vi "dht11.vi"() -> ()   [LabVIEW 2021]
panel:
  in  "Reset":bool
  out "HUMIDITY":dbl(knob) scale=0.0..100.0
  out "Thermometer":dbl(slide) scale=0.0..100.0
  in  "FAN":bool
  in  "PUMP":bool
  in  "VISA resource name":refnum<visa-resource-name>
  in  "stop":bool
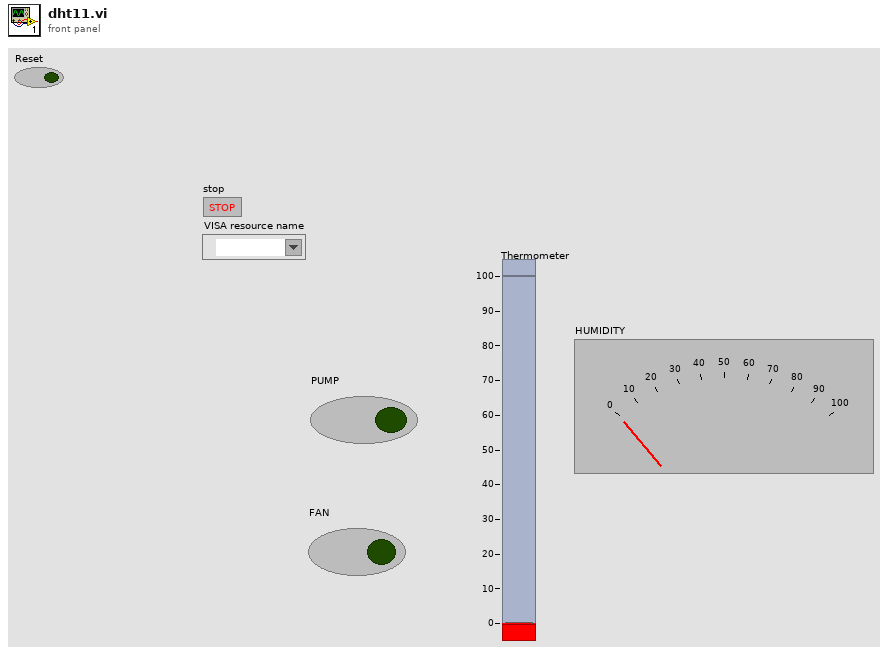
[diagram p1: front panel]
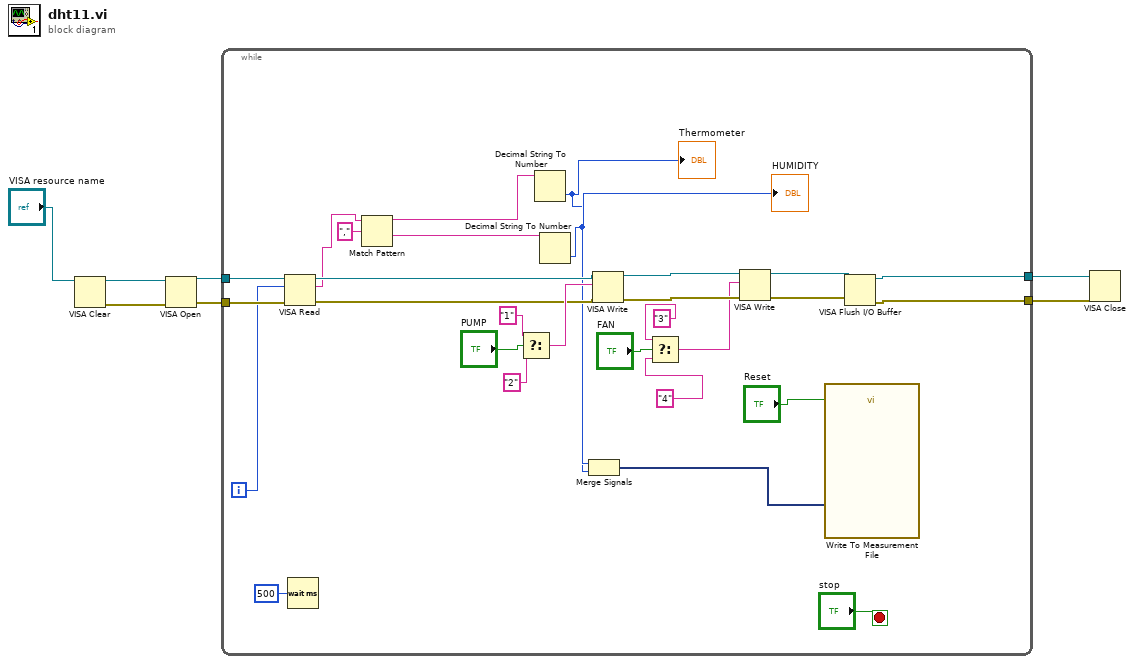
[diagram p0: block diagram]
diagram:
  n1 = VISA Clear(VISA resource name="VISA resource name") -> (VISA resource name out=w7:refnum<visa-resource-name>, error out=w6:errorcluster)  [unwired: 1 in]
  n2 = VISA Open(error in (no error)=w6, VISA resource name=w7) -> (VISA resource name=w5:refnum<visa-resource-name>, error out=w4:errorcluster)  [unwired: 3 in]
  n3 = while {
    tunnel: w5 -> [w36]
    tunnel: w4 -> [w35]
    tunnel: [w34] -> w3
    tunnel: [w33] -> w2
    i -> [w32]
    stop <- "stop" stop-if-true
    n4 = VISA Read(VISA resource name=w36, byte count=w32, error in (no error)=w35) -> (VISA resource name out=w17:refnum<visa-resource-name>, read buffer=w15:string, error out=w16:errorcluster)  [unwired: 1 out]
    n5 = Wait (ms)(milliseconds to wait=u32 500) -> ()  [unwired: 1 out]
    n6 = Match Pattern(string=w15, regular expression=",") -> (before substring=w13:string, after substring=w12:string)  [unwired: 1 in, 2 out]
    n7 = Select(t="1", s="PUMP", f="2") -> (s? t:f=w27:string)
    n8 = Decimal String To Number(string=w13) -> (number=w10:i32)  [unwired: 2 in, 1 out]
    "Thermometer" <- w10
    n9 = Decimal String To Number(string=w12) -> (number=w11:i32)  [unwired: 2 in, 1 out]
    "HUMIDITY" <- w11
    n10 = Merge Signals(w11, w10) -> (w9:dynamicdata)
    n11 = VISA Write(VISA resource name=w17, write buffer=w27, error in (no error)=w16) -> (VISA resource name out=w26:refnum<visa-resource-name>, error out=w24:errorcluster)  [unwired: 1 out]
    n12 = Select(t="3", s="FAN", f="4") -> (s? t:f=w21:string)
    n13 = VISA Write(VISA resource name=w26, write buffer=w21, error in (no error)=w24) -> (VISA resource name out=w25:refnum<visa-resource-name>, error out=w23:errorcluster)  [unwired: 1 out]
    n14 = call "Write To Measurement File"("Signals"=w9, "Reset"="Reset") -> ()  [unwired: 15 in, 3 out]
    n15 = VISA Flush I/O Buffer(VISA resource name=w25, error in (no error)=w23) -> (VISA resource name out=w34:refnum<visa-resource-name>, error out=w33:errorcluster)  [unwired: 1 in]
  }
  n16 = VISA Close(VISA resource name=w3, error in (no error)=w2) -> ()  [unwired: 1 out]
